vi "test_Split Registers by Direction.vi"(8 "error in (no error)":errorcluster, 11 "TestCase in":refnum<class "FPGA Addon Load And Parse Bitfile Unit Tests.lvclass">) -> (0 "error out":errorcluster, 3 "TestCase out":refnum<class "FPGA Addon Load And Parse Bitfile Unit Tests.lvclass">)   [LabVIEW 2018, in "FPGA Addon Load And Parse Bitfile Unit Tests.lvclass"]
uses:
  FPGA Addon Load And Parse Bitfile Unit Tests.lvclass
  Addon/Addon Shared/Types/Register Information.ctl
  Addon/Addon Shared/Types/FPGA Addon Data Type.ctl
  <vilib>/addons/_JKI Toolkits/VI Tester/TestCase.llb/TestCase.lvclass
  Addon/Addon System Explorer/FPGA Addon System Explorer.lvlib
  Addon/Addon Shared/FPGA Addon Shared.lvlib
  C:/Program Files (x86)/National Instruments/LabVIEW 2018/vi.lib/addons/_JKI Toolkits/VI Tester/TestCase.llb/TestCase.lvclass
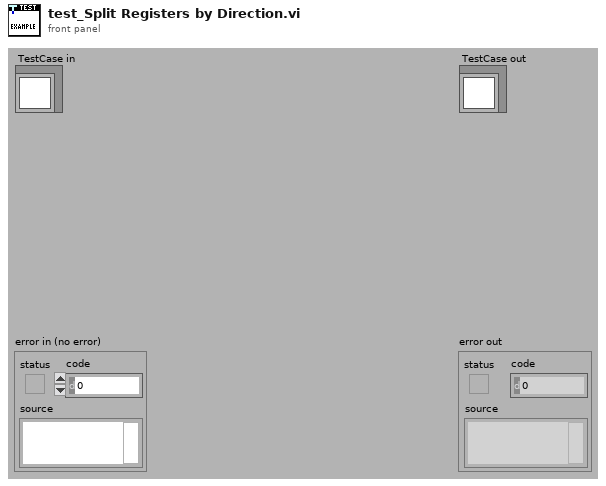
[diagram p1: front panel]
types:
  T1 = typedef "FPGA Addon Shared.lvlib/Register Information.ctl" = cluster{"Name":string, "Data Type":T2, "Default Value":variant, "Attributes":variant}
  T2 = typedef "FPGA Addon Shared.lvlib/FPGA Addon Data Type.ctl" = enum8{"<Null>", "I8", "I16", "I32", "I64", "U8", "U16", "U32", "U64", "SGL", "Boolean", "Analog PWM In Settings", "Analog PWM In", "Digital PWM In Settings", "Digital PWM In", "Digital PWM Out", "Sine Out", "FXP", "FXP+/-24.5", "FXP+/-16.5", "FXP+/-32.8", "FXP+/-64.32", "FXP+/-16.7", "FXP+/-20.5", "FXP+/-27.5", "FXP+/-32.16", "FXP+16.3", "FXP+18.3", "Digital Static In", "Digital Static Out", "Digital Static In Settings", "Digital WSS Out", "Quad Encoder Settings", "Quad Encoder In", "Group"}
  T3 = typedef "niFpgaBitfileStructure_VI.ctl" = cluster{"Name":string, "RegisterMap":T4[], "Icon":T9}
  T4 = typedef "nirviControlStructure.ctl" = cluster{"Name":string, "Hidden":bool, "Indicator":bool, "Flattened Type":string, "Grouping":cluster{"Grouped":bool, "Member Names":string[], "Member IDs":u32[]}, "Address":u32, "Size":u32, "Class":u32, "Internal":bool, "Typedef":T5, "ID":u32, "Bidirectional":bool, "Synchronous":bool, "Mechanical Action":T6, "Sub Controls":T7[], "Access May Timeout":bool, "Register Node":bool}
  T5 = typedef "nirviTypdefDescription.ctl" = cluster{"Typedef":bool, "Path":path}
  T6 = typedef "nirviMechanicalAction.ctl" = enum8{"Switch When Pressed", "Switch When Released", "Switch Until Released", "Latch When Pressed", "Latch When Released", "Latch Until Released"}
  T7 = typedef "nirviSubControlStructure.ctl" = cluster{"Name":string, "flattened Type":string, "Cluster Information":T8, "Typedef":T5}
  T8 = typedef "nirviClusterElementControl.ctl" = cluster{"Name Hierarchy":string[], "Item Order":u32[]}
  T9 = typedef "imagedata.ctl" = cluster{"image type":i32, "image depth":i32, "image":u8[], "mask":u8[], "colors":u32[], "Rectangle":cluster{"left":i16, "top":i16, "right":i16, "bottom":i16}}
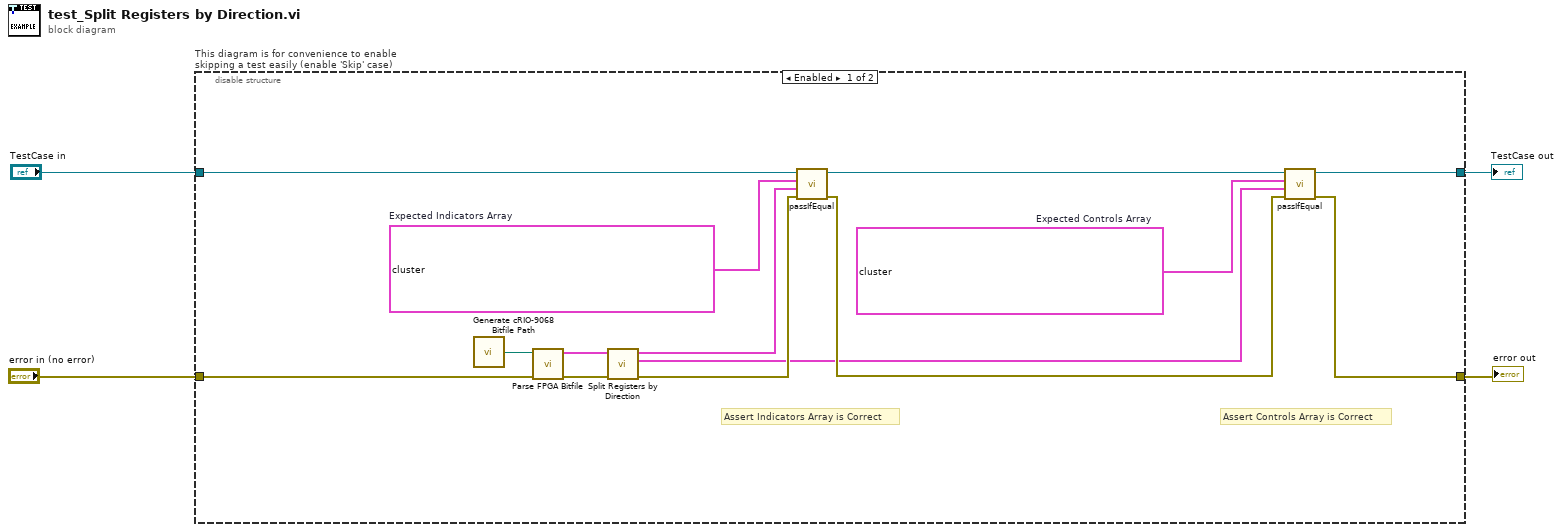
[diagram p0: block diagram]
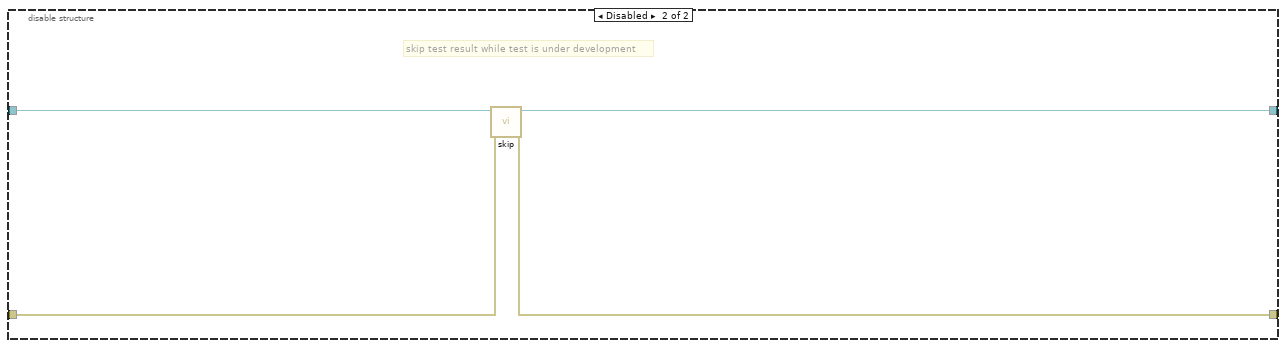
[diagram p2: hidden frame]
diagram:
  n1 = disable-structure "This diagram is for convenience to enable skipping a test easily (enable 'Skip' case)" shown="Enabled" {
    disable-tunnel: "TestCase in" -> [w18 w22]
    disable-tunnel: [w9 w20] -> w1
    disable-tunnel: [w12 w21] -> w3
    disable-tunnel: "error in (no error)" -> [w17 w19]
    frame Enabled {
      w5 = T1[] [{"Name"="Boolean", "Data Type"=enum."Boolean", "Default Value"=variant(dbl 0.0), "Attributes"=variant}, {"Name"="FXP16.3", "Data Type"=enum."FXP", "Default Value"=variant(fxp<+,16,3> 0.0), "Attributes"=variant(cluster{"FXP Representation":cluster{"Signed":bool, "Word Length":u32, "Integer Word Length":i32}, "FXP Range":cluster{"Range Min":dbl, "Range Max":dbl, "Delta":dbl}} {"FXP Representation"={"Signed"=FALSE, "Word Length"=16, "Integer Word Length"=3}, "FXP Range"={"Range Min"=0.0, "Range Max"=7.9998779296875, "Delta"=0.0001220703125}})}, {"Name"="FXP16.5", "Data Type"=enum."FXP", "Default Value"=variant(fxp<+/-,16,5> 0.0), "Attributes"=variant(cluster{"FXP Representation":cluster{"Signed":bool, "Word Length":u32, "Integer Word Length":i32}, "FXP Range":cluster{"Range Min":dbl, "Range Max":dbl, "Delta":dbl}} {"FXP Representation"={"Signed"=TRUE, "Word Length"=16, "Integer Word Length"=5}, "FXP Range"={"Range Min"=-16.0, "Range Max"=15.99951171875, "Delta"=0.00048828125}})}, {"Name"="FXP16.7", "Data Type"=enum."FXP", "Default Value"=variant(fxp<+/-,16,7> 0.0), "Attributes"=variant(cluster{"FXP Representation":cluster{"Signed":bool, "Word Length":u32, "Integer Word Length":i32}, "FXP Range":cluster{"Range Min":dbl, "Range Max":dbl, "Delta":dbl}} {"FXP Representation"={"Signed"=TRUE, "Word Length"=16, "Integer Word Length"=7}, "FXP Range"={"Range Min"=-64.0, "Range Max"=63.998046875, "Delta"=0.001953125}})}, {"Name"="FXP18.3", "Data Type"=enum."FXP", "Default Value"=variant(fxp<+,18,3> 0.0), "Attributes"=variant(cluster{"FXP Representation":cluster{"Signed":bool, "Word Length":u32, "Integer Word Length":i32}, "FXP Range":cluster{"Range Min":dbl, "Range Max":dbl, "Delta":dbl}} {"FXP Representation"={"Signed"=FALSE, "Word Length"=18, "Integer Word Length"=3}, "FXP Range"={"Range Min"=0.0, "Range Max"=7.999969482421875, "Delta"=3.0517578125e-05}})}, {"Name"="FXP20.5", "Data Type"=enum."FXP", "Default Value"=variant(fxp<+/-,20,5> 0.0), "Attributes"=variant(cluster{"FXP Representation":cluster{"Signed":bool, "Word Length":u32, "Integer Word Length":i32}, "FXP Range":cluster{"Range Min":dbl, "Range Max":dbl, "Delta":dbl}} {"FXP Representation"={"Signed"=TRUE, "Word Length"=20, "Integer Word Length"=5}, "FXP Range"={"Range Min"=-16.0, "Range Max"=15.999969482421875, "Delta"=3.0517578125e-05}})}, {"Name"="FXP24.5", "Data Type"=enum."FXP", "Default Value"=variant(fxp<+/-,24,5> 0.0), "Attributes"=variant(cluster{"FXP Representation":cluster{"Signed":bool, "Word Length":u32, "Integer Word Length":i32}, "FXP Range":cluster{"Range Min":dbl, "Range Max":dbl, "Delta":dbl}} {"FXP Representation"={"Signed"=TRUE, "Word Length"=24, "Integer Word Length"=5}, "FXP Range"={"Range Min"=-16.0, "Range Max"=15.999998092651367, "Delta"=1.9073486328125e-06}})}, {"Name"="FXP27.5", "Data Type"=enum."FXP", "Default Value"=variant(fxp<+/-,27,5> 0.0), "Attributes"=variant(cluster{"FXP Representation":cluster{"Signed":bool, "Word Length":u32, "Integer Word Length":i32}, "FXP Range":cluster{"Range Min":dbl, "Range Max":dbl, "Delta":dbl}} {"FXP Representation"={"Signed"=TRUE, "Word Length"=27, "Integer Word Length"=5}, "FXP Range"={"Range Min"=-16.0, "Range Max"=15.999999761581421, "Delta"=2.384185791015625e-07}})}, {"Name"="FXP32.16", "Data Type"=enum."FXP", "Default Value"=variant(fxp<+/-,32,16> 0.0), "Attributes"=variant(cluster{"FXP Representation":cluster{"Signed":bool, "Word Length":u32, "Integer Word Length":i32}, "FXP Range":cluster{"Range Min":dbl, "Range Max":dbl, "Delta":dbl}} {"FXP Representation"={"Signed"=TRUE, "Word Length"=32, "Integer Word Length"=16}, "FXP Range"={"Range Min"=-32768.0, "Range Max"=32767.99998474121, "Delta"=1.52587890625e-05}})}, {"Name"="FXP32.8", "Data Type"=enum."FXP", "Default Value"=variant(fxp<+/-,32,8> 0.0), "Attributes"=variant(cluster{"FXP Representation":cluster{"Signed":bool, "Word Length":u32, "Integer Word Length":i32}, "FXP Range":cluster{"Range Min":dbl, "Range Max":dbl, "Delta":dbl}} {"FXP Representation"={"Signed"=TRUE, "Word Length"=32, "Integer Word Length"=8}, "FXP Range"={"Range Min"=-128.0, "Range Max"=127.99999994039536, "Delta"=5.960464477539063e-08}})}, {"Name"="FXP64.32", "Data Type"=enum."FXP", "Default Value"=variant(fxp<+/-,64,32> 0.0), "Attributes"=variant(cluster{"FXP Representation":cluster{"Signed":bool, "Word Length":u32, "Integer Word Length":i32}, "FXP Range":cluster{"Range Min":dbl, "Range Max":dbl, "Delta":dbl}} {"FXP Representation"={"Signed"=TRUE, "Word Length"=64, "Integer Word Length"=32}, "FXP Range"={"Range Min"=-2147483648.0, "Range Max"=2147483648.0, "Delta"=2.3283064365386963e-10}})}, {"Name"="Group1.I16", "Data Type"=enum."I16", "Default Value"=variant(dbl 0.0), "Attributes"=variant}, {"Name"="Group1.I32", "Data Type"=enum."I32", "Default Value"=variant(dbl 0.0), "Attributes"=variant}, {"Name"="Group1.I64", "Data Type"=enum."I64", "Default Value"=variant(dbl 0.0), "Attributes"=variant}, {"Name"="Group1.I8", "Data Type"=enum."I8", "Default Value"=variant(dbl 0.0), "Attributes"=variant}, {"Name"="Group1.SGL", "Data Type"=enum."SGL", "Default Value"=variant(dbl 0.0), "Attributes"=variant}, {"Name"="Group1.U16", "Data Type"=enum."U16", "Default Value"=variant(dbl 0.0), "Attributes"=variant}, {"Name"="Group1.U32", "Data Type"=enum."U32", "Default Value"=variant(dbl 0.0), "Attributes"=variant}, {"Name"="Group1.U64", "Data Type"=enum."U64", "Default Value"=variant(dbl 0.0), "Attributes"=variant}, {"Name"="Group1.U8", "Data Type"=enum."U8", "Default Value"=variant(dbl 0.0), "Attributes"=variant}, {"Name"="Group2.Boolean", "Data Type"=enum."Boolean", "Default Value"=variant(dbl 0.0), "Attributes"=variant}, {"Name"="Group2.FXP16.3", "Data Type"=enum."FXP", "Default Value"=variant(fxp<+,16,3> 0.0), "Attributes"=variant(cluster{"FXP Representation":cluster{"Signed":bool, "Word Length":u32, "Integer Word Length":i32}, "FXP Range":cluster{"Range Min":dbl, "Range Max":dbl, "Delta":dbl}} {"FXP Representation"={"Signed"=FALSE, "Word Length"=16, "Integer Word Length"=3}, "FXP Range"={"Range Min"=0.0, "Range Max"=7.9998779296875, "Delta"=0.0001220703125}})}, {"Name"="Group2.FXP16.5", "Data Type"=enum."FXP", "Default Value"=variant(fxp<+/-,16,5> 0.0), "Attributes"=variant(cluster{"FXP Representation":cluster{"Signed":bool, "Word Length":u32, "Integer Word Length":i32}, "FXP Range":cluster{"Range Min":dbl, "Range Max":dbl, "Delta":dbl}} {"FXP Representation"={"Signed"=TRUE, "Word Length"=16, "Integer Word Length"=5}, "FXP Range"={"Range Min"=-16.0, "Range Max"=15.99951171875, "Delta"=0.00048828125}})}, {"Name"="Group2.FXP16.7", "Data Type"=enum."FXP", "Default Value"=variant(fxp<+/-,16,7> 0.0), "Attributes"=variant(cluster{"FXP Representation":cluster{"Signed":bool, "Word Length":u32, "Integer Word Length":i32}, "FXP Range":cluster{"Range Min":dbl, "Range Max":dbl, "Delta":dbl}} {"FXP Representation"={"Signed"=TRUE, "Word Length"=16, "Integer Word Length"=7}, "FXP Range"={"Range Min"=-64.0, "Range Max"=63.998046875, "Delta"=0.001953125}})}, {"Name"="Group2.FXP18.3", "Data Type"=enum."FXP", "Default Value"=variant(fxp<+,18,3> 0.0), "Attributes"=variant(cluster{"FXP Representation":cluster{"Signed":bool, "Word Length":u32, "Integer Word Length":i32}, "FXP Range":cluster{"Range Min":dbl, "Range Max":dbl, "Delta":dbl}} {"FXP Representation"={"Signed"=FALSE, "Word Length"=18, "Integer Word Length"=3}, "FXP Range"={"Range Min"=0.0, "Range Max"=7.999969482421875, "Delta"=3.0517578125e-05}})}, {"Name"="Group2.FXP20.5", "Data Type"=enum."FXP", "Default Value"=variant(fxp<+/-,20,5> 0.0), "Attributes"=variant(cluster{"FXP Representation":cluster{"Signed":bool, "Word Length":u32, "Integer Word Length":i32}, "FXP Range":cluster{"Range Min":dbl, "Range Max":dbl, "Delta":dbl}} {"FXP Representation"={"Signed"=TRUE, "Word Length"=20, "Integer Word Length"=5}, "FXP Range"={"Range Min"=-16.0, "Range Max"=15.999969482421875, "Delta"=3.0517578125e-05}})}, {"Name"="Group2.FXP24.5", "Data Type"=enum."FXP", "Default Value"=variant(fxp<+/-,24,5> 0.0), "Attributes"=variant(cluster{"FXP Representation":cluster{"Signed":bool, "Word Length":u32, "Integer Word Length":i32}, "FXP Range":cluster{"Range Min":dbl, "Range Max":dbl, "Delta":dbl}} {"FXP Representation"={"Signed"=TRUE, "Word Length"=24, "Integer Word Length"=5}, "FXP Range"={"Range Min"=-16.0, "Range Max"=15.999998092651367, "Delta"=1.9073486328125e-06}})}, {"Name"="Group2.FXP27.5", "Data Type"=enum."FXP", "Default Value"=variant(fxp<+/-,27,5> 0.0), "Attributes"=variant(cluster{"FXP Representation":cluster{"Signed":bool, "Word Length":u32, "Integer Word Length":i32}, "FXP Range":cluster{"Range Min":dbl, "Range Max":dbl, "Delta":dbl}} {"FXP Representation"={"Signed"=TRUE, "Word Length"=27, "Integer Word Length"=5}, "FXP Range"={"Range Min"=-16.0, "Range Max"=15.999999761581421, "Delta"=2.384185791015625e-07}})}, {"Name"="Group2.FXP32.16", "Data Type"=enum."FXP", "Default Value"=variant(fxp<+/-,32,16> 0.0), "Attributes"=variant(cluster{"FXP Representation":cluster{"Signed":bool, "Word Length":u32, "Integer Word Length":i32}, "FXP Range":cluster{"Range Min":dbl, "Range Max":dbl, "Delta":dbl}} {"FXP Representation"={"Signed"=TRUE, "Word Length"=32, "Integer Word Length"=16}, "FXP Range"={"Range Min"=-32768.0, "Range Max"=32767.99998474121, "Delta"=1.52587890625e-05}})}, {"Name"="Group2.FXP32.8", "Data Type"=enum."FXP", "Default Value"=variant(fxp<+/-,32,8> 0.0), "Attributes"=variant(cluster{"FXP Representation":cluster{"Signed":bool, "Word Length":u32, "Integer Word Length":i32}, "FXP Range":cluster{"Range Min":dbl, "Range Max":dbl, "Delta":dbl}} {"FXP Representation"={"Signed"=TRUE, "Word Length"=32, "Integer Word Length"=8}, "FXP Range"={"Range Min"=-128.0, "Range Max"=127.99999994039536, "Delta"=5.960464477539063e-08}})}, {"Name"="Group2.FXP64.32", "Data Type"=enum."FXP", "Default Value"=variant(fxp<+/-,64,32> 0.0), "Attributes"=variant(cluster{"FXP Representation":cluster{"Signed":bool, "Word Length":u32, "Integer Word Length":i32}, "FXP Range":cluster{"Range Min":dbl, "Range Max":dbl, "Delta":dbl}} {"FXP Representation"={"Signed"=TRUE, "Word Length"=64, "Integer Word Length"=32}, "FXP Range"={"Range Min"=-2147483648.0, "Range Max"=2147483648.0, "Delta"=2.3283064365386963e-10}})}, {"Name"="I16", "Data Type"=enum."I16", "Default Value"=variant(dbl 0.0), "Attributes"=variant}, {"Name"="I32", "Data Type"=enum."I32", "Default Value"=variant(dbl 0.0), "Attributes"=variant}, {"Name"="I64", "Data Type"=enum."I64", "Default Value"=variant(dbl 0.0), "Attributes"=variant}, {"Name"="I8", "Data Type"=enum."I8", "Default Value"=variant(dbl 0.0), "Attributes"=variant}, {"Name"="SGL", "Data Type"=enum."SGL", "Default Value"=variant(dbl 0.0), "Attributes"=variant}, {"Name"="U16", "Data Type"=enum."U16", "Default Value"=variant(dbl 0.0), "Attributes"=variant}, {"Name"="U32", "Data Type"=enum."U32", "Default Value"=variant(dbl 0.0), "Attributes"=variant}, {"Name"="U64", "Data Type"=enum."U64", "Default Value"=variant(dbl 0.0), "Attributes"=variant}, {"Name"="U8", "Data Type"=enum."U8", "Default Value"=variant(dbl 0.0), "Attributes"=variant}]  # Expected Controls Array
      w6 = T1[] [{"Name"="Boolean out", "Data Type"=enum."Boolean", "Default Value"=variant(dbl 0.0), "Attributes"=variant}, {"Name"="FXP16.3 out", "Data Type"=enum."FXP", "Default Value"=variant(fxp<+,16,3> 0.0), "Attributes"=variant(cluster{"FXP Representation":cluster{"Signed":bool, "Word Length":u32, "Integer Word Length":i32}, "FXP Range":cluster{"Range Min":dbl, "Range Max":dbl, "Delta":dbl}} {"FXP Representation"={"Signed"=FALSE, "Word Length"=16, "Integer Word Length"=3}, "FXP Range"={"Range Min"=0.0, "Range Max"=7.9998779296875, "Delta"=0.0001220703125}})}, {"Name"="FXP16.5 out", "Data Type"=enum."FXP", "Default Value"=variant(fxp<+/-,16,5> 0.0), "Attributes"=variant(cluster{"FXP Representation":cluster{"Signed":bool, "Word Length":u32, "Integer Word Length":i32}, "FXP Range":cluster{"Range Min":dbl, "Range Max":dbl, "Delta":dbl}} {"FXP Representation"={"Signed"=TRUE, "Word Length"=16, "Integer Word Length"=5}, "FXP Range"={"Range Min"=-16.0, "Range Max"=15.99951171875, "Delta"=0.00048828125}})}, {"Name"="FXP16.7 out", "Data Type"=enum."FXP", "Default Value"=variant(fxp<+/-,16,7> 0.0), "Attributes"=variant(cluster{"FXP Representation":cluster{"Signed":bool, "Word Length":u32, "Integer Word Length":i32}, "FXP Range":cluster{"Range Min":dbl, "Range Max":dbl, "Delta":dbl}} {"FXP Representation"={"Signed"=TRUE, "Word Length"=16, "Integer Word Length"=7}, "FXP Range"={"Range Min"=-64.0, "Range Max"=63.998046875, "Delta"=0.001953125}})}, {"Name"="FXP18.3 out", "Data Type"=enum."FXP", "Default Value"=variant(fxp<+,18,3> 0.0), "Attributes"=variant(cluster{"FXP Representation":cluster{"Signed":bool, "Word Length":u32, "Integer Word Length":i32}, "FXP Range":cluster{"Range Min":dbl, "Range Max":dbl, "Delta":dbl}} {"FXP Representation"={"Signed"=FALSE, "Word Length"=18, "Integer Word Length"=3}, "FXP Range"={"Range Min"=0.0, "Range Max"=7.999969482421875, "Delta"=3.0517578125e-05}})}, {"Name"="FXP20.5 out", "Data Type"=enum."FXP", "Default Value"=variant(fxp<+/-,20,5> 0.0), "Attributes"=variant(cluster{"FXP Representation":cluster{"Signed":bool, "Word Length":u32, "Integer Word Length":i32}, "FXP Range":cluster{"Range Min":dbl, "Range Max":dbl, "Delta":dbl}} {"FXP Representation"={"Signed"=TRUE, "Word Length"=20, "Integer Word Length"=5}, "FXP Range"={"Range Min"=-16.0, "Range Max"=15.999969482421875, "Delta"=3.0517578125e-05}})}, {"Name"="FXP24.5 out", "Data Type"=enum."FXP", "Default Value"=variant(fxp<+/-,24,5> 0.0), "Attributes"=variant(cluster{"FXP Representation":cluster{"Signed":bool, "Word Length":u32, "Integer Word Length":i32}, "FXP Range":cluster{"Range Min":dbl, "Range Max":dbl, "Delta":dbl}} {"FXP Representation"={"Signed"=TRUE, "Word Length"=24, "Integer Word Length"=5}, "FXP Range"={"Range Min"=-16.0, "Range Max"=15.999998092651367, "Delta"=1.9073486328125e-06}})}, {"Name"="FXP27.5 out", "Data Type"=enum."FXP", "Default Value"=variant(fxp<+/-,27,5> 0.0), "Attributes"=variant(cluster{"FXP Representation":cluster{"Signed":bool, "Word Length":u32, "Integer Word Length":i32}, "FXP Range":cluster{"Range Min":dbl, "Range Max":dbl, "Delta":dbl}} {"FXP Representation"={"Signed"=TRUE, "Word Length"=27, "Integer Word Length"=5}, "FXP Range"={"Range Min"=-16.0, "Range Max"=15.999999761581421, "Delta"=2.384185791015625e-07}})}, {"Name"="FXP32.16 out", "Data Type"=enum."FXP", "Default Value"=variant(fxp<+/-,32,16> 0.0), "Attributes"=variant(cluster{"FXP Representation":cluster{"Signed":bool, "Word Length":u32, "Integer Word Length":i32}, "FXP Range":cluster{"Range Min":dbl, "Range Max":dbl, "Delta":dbl}} {"FXP Representation"={"Signed"=TRUE, "Word Length"=32, "Integer Word Length"=16}, "FXP Range"={"Range Min"=-32768.0, "Range Max"=32767.99998474121, "Delta"=1.52587890625e-05}})}, {"Name"="FXP32.8 out", "Data Type"=enum."FXP", "Default Value"=variant(fxp<+/-,32,8> 0.0), "Attributes"=variant(cluster{"FXP Representation":cluster{"Signed":bool, "Word Length":u32, "Integer Word Length":i32}, "FXP Range":cluster{"Range Min":dbl, "Range Max":dbl, "Delta":dbl}} {"FXP Representation"={"Signed"=TRUE, "Word Length"=32, "Integer Word Length"=8}, "FXP Range"={"Range Min"=-128.0, "Range Max"=127.99999994039536, "Delta"=5.960464477539063e-08}})}, {"Name"="FXP64.32 out", "Data Type"=enum."FXP", "Default Value"=variant(fxp<+/-,64,32> 0.0), "Attributes"=variant(cluster{"FXP Representation":cluster{"Signed":bool, "Word Length":u32, "Integer Word Length":i32}, "FXP Range":cluster{"Range Min":dbl, "Range Max":dbl, "Delta":dbl}} {"FXP Representation"={"Signed"=TRUE, "Word Length"=64, "Integer Word Length"=32}, "FXP Range"={"Range Min"=-2147483648.0, "Range Max"=2147483648.0, "Delta"=2.3283064365386963e-10}})}, {"Name"="Fast timeout", "Data Type"=enum."Boolean", "Default Value"=variant(dbl 0.0), "Attributes"=variant}, {"Name"="Fast timeout 2", "Data Type"=enum."Boolean", "Default Value"=variant(dbl 0.0), "Attributes"=variant}, {"Name"="Fast timeout 3", "Data Type"=enum."Boolean", "Default Value"=variant(dbl 0.0), "Attributes"=variant}, {"Name"="Group1.I16 out", "Data Type"=enum."I16", "Default Value"=variant(dbl 0.0), "Attributes"=variant}, {"Name"="Group1.I32 out", "Data Type"=enum."I32", "Default Value"=variant(dbl 0.0), "Attributes"=variant}, {"Name"="Group1.I64 out", "Data Type"=enum."I64", "Default Value"=variant(dbl 0.0), "Attributes"=variant}, {"Name"="Group1.I8 out", "Data Type"=enum."I8", "Default Value"=variant(dbl 0.0), "Attributes"=variant}, {"Name"="Group1.SGL out", "Data Type"=enum."SGL", "Default Value"=variant(dbl 0.0), "Attributes"=variant}, {"Name"="Group1.U16 out", "Data Type"=enum."U16", "Default Value"=variant(dbl 0.0), "Attributes"=variant}, {"Name"="Group1.U32 out", "Data Type"=enum."U32", "Default Value"=variant(dbl 0.0), "Attributes"=variant}, {"Name"="Group1.U64 out", "Data Type"=enum."U64", "Default Value"=variant(dbl 0.0), "Attributes"=variant}, {"Name"="Group1.U8 out", "Data Type"=enum."U8", "Default Value"=variant(dbl 0.0), "Attributes"=variant}, {"Name"="Group2.Boolean out", "Data Type"=enum."Boolean", "Default Value"=variant(dbl 0.0), "Attributes"=variant}, {"Name"="Group2.FXP16.3 out", "Data Type"=enum."FXP", "Default Value"=variant(fxp<+,16,3> 0.0), "Attributes"=variant(cluster{"FXP Representation":cluster{"Signed":bool, "Word Length":u32, "Integer Word Length":i32}, "FXP Range":cluster{"Range Min":dbl, "Range Max":dbl, "Delta":dbl}} {"FXP Representation"={"Signed"=FALSE, "Word Length"=16, "Integer Word Length"=3}, "FXP Range"={"Range Min"=0.0, "Range Max"=7.9998779296875, "Delta"=0.0001220703125}})}, {"Name"="Group2.FXP16.5 out", "Data Type"=enum."FXP", "Default Value"=variant(fxp<+/-,16,5> 0.0), "Attributes"=variant(cluster{"FXP Representation":cluster{"Signed":bool, "Word Length":u32, "Integer Word Length":i32}, "FXP Range":cluster{"Range Min":dbl, "Range Max":dbl, "Delta":dbl}} {"FXP Representation"={"Signed"=TRUE, "Word Length"=16, "Integer Word Length"=5}, "FXP Range"={"Range Min"=-16.0, "Range Max"=15.99951171875, "Delta"=0.00048828125}})}, {"Name"="Group2.FXP16.7 out", "Data Type"=enum."FXP", "Default Value"=variant(fxp<+/-,16,7> 0.0), "Attributes"=variant(cluster{"FXP Representation":cluster{"Signed":bool, "Word Length":u32, "Integer Word Length":i32}, "FXP Range":cluster{"Range Min":dbl, "Range Max":dbl, "Delta":dbl}} {"FXP Representation"={"Signed"=TRUE, "Word Length"=16, "Integer Word Length"=7}, "FXP Range"={"Range Min"=-64.0, "Range Max"=63.998046875, "Delta"=0.001953125}})}, {"Name"="Group2.FXP18.3 out", "Data Type"=enum."FXP", "Default Value"=variant(fxp<+,18,3> 0.0), "Attributes"=variant(cluster{"FXP Representation":cluster{"Signed":bool, "Word Length":u32, "Integer Word Length":i32}, "FXP Range":cluster{"Range Min":dbl, "Range Max":dbl, "Delta":dbl}} {"FXP Representation"={"Signed"=FALSE, "Word Length"=18, "Integer Word Length"=3}, "FXP Range"={"Range Min"=0.0, "Range Max"=7.999969482421875, "Delta"=3.0517578125e-05}})}, {"Name"="Group2.FXP20.5 out", "Data Type"=enum."FXP", "Default Value"=variant(fxp<+/-,20,5> 0.0), "Attributes"=variant(cluster{"FXP Representation":cluster{"Signed":bool, "Word Length":u32, "Integer Word Length":i32}, "FXP Range":cluster{"Range Min":dbl, "Range Max":dbl, "Delta":dbl}} {"FXP Representation"={"Signed"=TRUE, "Word Length"=20, "Integer Word Length"=5}, "FXP Range"={"Range Min"=-16.0, "Range Max"=15.999969482421875, "Delta"=3.0517578125e-05}})}, {"Name"="Group2.FXP24.5 out", "Data Type"=enum."FXP", "Default Value"=variant(fxp<+/-,24,5> 0.0), "Attributes"=variant(cluster{"FXP Representation":cluster{"Signed":bool, "Word Length":u32, "Integer Word Length":i32}, "FXP Range":cluster{"Range Min":dbl, "Range Max":dbl, "Delta":dbl}} {"FXP Representation"={"Signed"=TRUE, "Word Length"=24, "Integer Word Length"=5}, "FXP Range"={"Range Min"=-16.0, "Range Max"=15.999998092651367, "Delta"=1.9073486328125e-06}})}, {"Name"="Group2.FXP27.5 out", "Data Type"=enum."FXP", "Default Value"=variant(fxp<+/-,27,5> 0.0), "Attributes"=variant(cluster{"FXP Representation":cluster{"Signed":bool, "Word Length":u32, "Integer Word Length":i32}, "FXP Range":cluster{"Range Min":dbl, "Range Max":dbl, "Delta":dbl}} {"FXP Representation"={"Signed"=TRUE, "Word Length"=27, "Integer Word Length"=5}, "FXP Range"={"Range Min"=-16.0, "Range Max"=15.999999761581421, "Delta"=2.384185791015625e-07}})}, {"Name"="Group2.FXP32.16 out", "Data Type"=enum."FXP", "Default Value"=variant(fxp<+/-,32,16> 0.0), "Attributes"=variant(cluster{"FXP Representation":cluster{"Signed":bool, "Word Length":u32, "Integer Word Length":i32}, "FXP Range":cluster{"Range Min":dbl, "Range Max":dbl, "Delta":dbl}} {"FXP Representation"={"Signed"=TRUE, "Word Length"=32, "Integer Word Length"=16}, "FXP Range"={"Range Min"=-32768.0, "Range Max"=32767.99998474121, "Delta"=1.52587890625e-05}})}, {"Name"="Group2.FXP32.8 out", "Data Type"=enum."FXP", "Default Value"=variant(fxp<+/-,32,8> 0.0), "Attributes"=variant(cluster{"FXP Representation":cluster{"Signed":bool, "Word Length":u32, "Integer Word Length":i32}, "FXP Range":cluster{"Range Min":dbl, "Range Max":dbl, "Delta":dbl}} {"FXP Representation"={"Signed"=TRUE, "Word Length"=32, "Integer Word Length"=8}, "FXP Range"={"Range Min"=-128.0, "Range Max"=127.99999994039536, "Delta"=5.960464477539063e-08}})}, {"Name"="Group2.FXP64.32 out", "Data Type"=enum."FXP", "Default Value"=variant(fxp<+/-,64,32> 0.0), "Attributes"=variant(cluster{"FXP Representation":cluster{"Signed":bool, "Word Length":u32, "Integer Word Length":i32}, "FXP Range":cluster{"Range Min":dbl, "Range Max":dbl, "Delta":dbl}} {"FXP Representation"={"Signed"=TRUE, "Word Length"=64, "Integer Word Length"=32}, "FXP Range"={"Range Min"=-2147483648.0, "Range Max"=2147483648.0, "Delta"=2.3283064365386963e-10}})}, {"Name"="I16 out", "Data Type"=enum."I16", "Default Value"=variant(dbl 0.0), "Attributes"=variant}, {"Name"="I32 out", "Data Type"=enum."I32", "Default Value"=variant(dbl 0.0), "Attributes"=variant}, {"Name"="I64 out", "Data Type"=enum."I64", "Default Value"=variant(dbl 0.0), "Attributes"=variant}, {"Name"="I8 out", "Data Type"=enum."I8", "Default Value"=variant(dbl 0.0), "Attributes"=variant}, {"Name"="Med timeout", "Data Type"=enum."Boolean", "Default Value"=variant(dbl 0.0), "Attributes"=variant}, {"Name"="SGL out", "Data Type"=enum."SGL", "Default Value"=variant(dbl 0.0), "Attributes"=variant}, {"Name"="Slow timeout", "Data Type"=enum."Boolean", "Default Value"=variant(dbl 0.0), "Attributes"=variant}, {"Name"="U16 out", "Data Type"=enum."U16", "Default Value"=variant(dbl 0.0), "Attributes"=variant}, {"Name"="U32 out", "Data Type"=enum."U32", "Default Value"=variant(dbl 0.0), "Attributes"=variant}, {"Name"="U64 out", "Data Type"=enum."U64", "Default Value"=variant(dbl 0.0), "Attributes"=variant}, {"Name"="U8 out", "Data Type"=enum."U8", "Default Value"=variant(dbl 0.0), "Attributes"=variant}]  # Expected Indicators Array
      # "Assert Controls Array is Correct"
      # "Assert Indicators Array is Correct"
      n2 = call "Generate cRIO-9068 Bitfile Path.vi"() -> ("Bitfile Path"=w8:path)
      n3 = call "Parse FPGA Bitfile.vi"("error in (no error)"=w17, "Path"=w8) -> ("error out"=w16:errorcluster, "vi info"=w15:T3)  [unwired: 7 in, 1 out]
      n4 = call "Split Registers by Direction.vi"("error in"=w16, "vi info"=w15) -> ("error out"=w14:errorcluster, "Controls"=w7:T1[], "Indicator"=w13:T1[])  [unwired: 7 in]
      n5 = call-dynamic "passIfEqual.vi"("error in (no error)"=w14, "y"=w13, "x"=w6, "TestCase in"=w18) -> ("error out"=w11:errorcluster, "TestCase out"=w10:refnum<class "FPGA Addon Load And Parse Bitfile Unit Tests.lvclass">)  [unwired: 6 in]
      n6 = call-dynamic "passIfEqual.vi"("error in (no error)"=w11, "y"=w7, "x"=w5, "TestCase in"=w10) -> ("error out"=w12:errorcluster, "TestCase out"=w9:refnum<class "FPGA Addon Load And Parse Bitfile Unit Tests.lvclass">)  [unwired: 6 in]
    }
    frame Disabled {
      # "skip test result while test is under development"
      n7 = call <vilib>:"skip.vi"("error in (no error)"=w19, "TestCase in"=w22) -> ("error out"=w21:errorcluster, "TestCase out"=w20:refnum<class "FPGA Addon Load And Parse Bitfile Unit Tests.lvclass">)  [unwired: 8 in]
    }
  }
  "error out" <- w3
  "TestCase out" <- w1
